vi "SSDPPacket.vi"(10 "data":string, 11 "getMethods":u16(ring) items=["getHost()", "getCacheControl()", "getLocation()", "getMAN()", "getST()", "getNT()", "getNTS()", "getServer()", "getUSN()", "getMX()"]) -> (3 "value":string)   [LabVIEW 2010]
uses:
  <vilib>/Utility/error.llb/whitespace.ctl
  <vilib>/regexp/Match Regular Expression.xnode
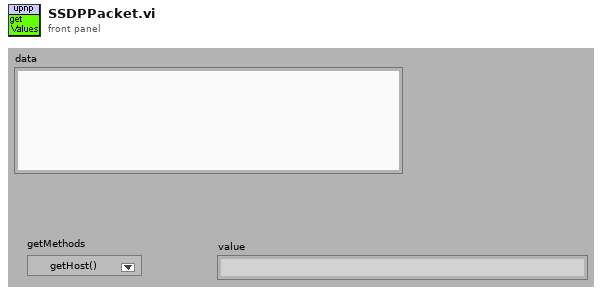
[diagram p1: front panel]
types:
  T1 = typedef "whitespace.ctl" = u16
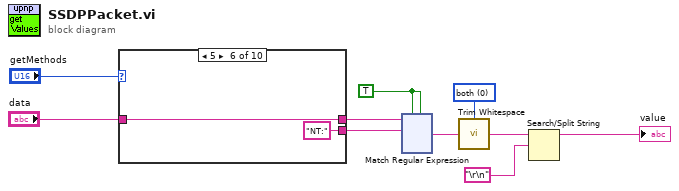
[diagram p0: block diagram]
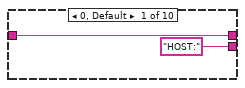
[diagram p2: hidden frame]
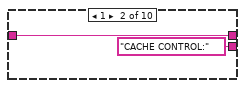
[diagram p3: hidden frame]
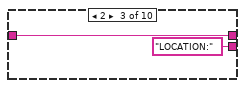
[diagram p4: hidden frame]
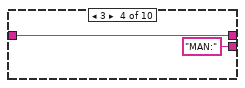
[diagram p5: hidden frame]
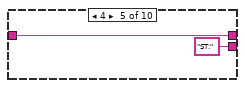
[diagram p6: hidden frame]
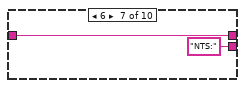
[diagram p7: hidden frame]
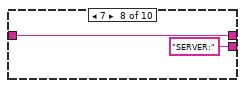
[diagram p8: hidden frame]
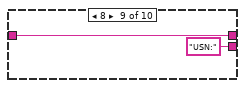
[diagram p9: hidden frame]
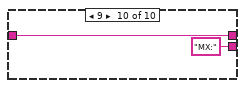
[diagram p10: hidden frame]
diagram:
  w1 = T1 0 items=["both", "start of string", "end of string"] ("location (both)")
  w4 = TRUE ("multiline? (F)")
  n1 = case shown="5" "getMethods" {
    tunnel: "data" -> [w12 w14 w16 w18 w20 w22 w24 w26 w28 w30]
    tunnel: [w12 w14 w16 w18 w20 w22 w24 w26 w28 w30] -> w7
    tunnel: ["HOST:" ("search string") "CACHE CONTROL:" ("search string") "LOCATION:" ("search string") "MAN:" ("search string") "ST:" ("search string") "NT:" ("search string") "NTS:" ("search string") "SERVER:" ("search string") "USN:" ("search string") "MX:" ("search string")] -> w6
    frame 0, Default {
    }
    frame 1 {
    }
    frame 2 {
    }
    frame 3 {
    }
    frame 4 {
    }
    frame 5 {
    }
    frame 6 {
    }
    frame 7 {
    }
    frame 8 {
    }
    frame 9 {
    }
  }
  n2 = xnode "Match Regular Expression"("input string"=w7, "regular expression"=w6, "ignore case? (F)"=w4, "multiline? (F)"=w4) -> ("after match"=w3:string)  [unwired: 2 in, 4 out]
  n3 = call <vilib>:"Trim Whitespace.vi"("string"=w3, "location (both)"=w1) -> ("trimmed string"=w2:string)
  n4 = Search/Split String(string=w2, search string/char (-)="\r\n") -> (substring before match=→"value":string)  [unwired: 3 out]
